vi "ADS1015 Config Formatter.vi"(11 "ADS1015 Config Options":T1 {"Comparator Queue & Disable" items=["Assert after one conversion", "Assert after two conversions", "Assert after four conversions", "Comparator disabled"]; "Latching Comparator" items=["Non-latching", "Latching"]; "Comparator Polarity" items=["Active Low", "Active High"]; "Comparator Mode" items=["Traditional Comparator w/ hysteresis", "Window Comparator"]; "Sampling Rate" items=["128SPS", "250SPS", "490SPS", "920SPS", "1600SPS", "2400SPS", "3300SPS"]; "Sampling Mode" items=["Continuous Conversion", "Single-shot (Low Power)"]; "Expected Range (Programmable Gain Amplifier)" items=["+/-6.144V", "+/-4.096V", "+/-2.048V", "+/-1.024V", "+/-0.512V", "+/-0.256V"]; "Channel" items=["Differential: Ch 0&1", "Differential: Ch 0&3", "Differential: Ch 1&3", "Differential: Ch 2&3", "Single Ended: Ch 0", "Single Ended: Ch 1", "Single Ended: Ch 2", "Single Ended: Ch 3"]}) -> (3 "Config Command":u16=4096 format="%.0x")   [LabVIEW 2014]
uses:
  ADS1015 Config Options.ctl
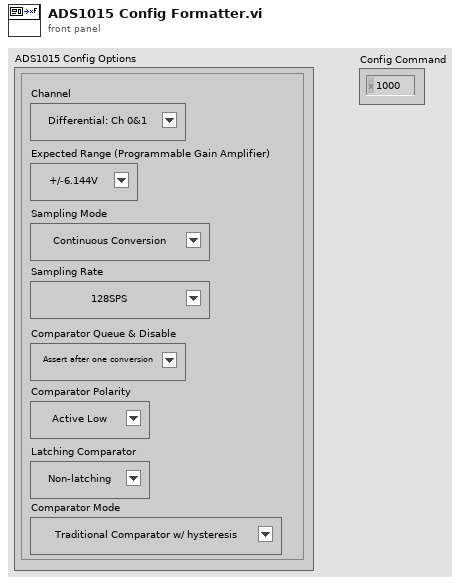
[diagram p1: front panel]
types:
  T1 = typedef "ADS1015 Config Options.ctl" = cluster{"Channel":u8, "Expected Range (Programmable Gain Amplifier)":u8, "Sampling Mode":u8, "Sampling Rate":u8, "Comparator Mode":u8, "Comparator Polarity":u8, "Latching Comparator":u8, "Comparator Queue & Disable":u8}
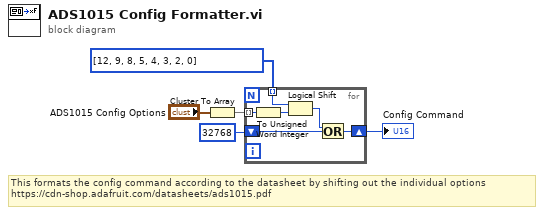
[diagram p0: block diagram]
diagram:
  # "This formats the config command according to the datasheet by shifting out the individual options\nhttps://cdn-shop.adafruit.com/datasheets/ads1015.pdf"
  n1 = Cluster To Array(cluster="ADS1015 Config Options") -> (array=w4:u8[])
  n2 = for {
    tunnel: w4 -> [w11] mode=indexing
    tunnel: i16[] [12, 9, 8, 5, 4, 3, 2, 0] -> [w10] mode=indexing
    shift-right: [w8] -> w1
    shift-left: u16 32768 -> [w7]
    n3 = To Unsigned Word Integer(number=w11) -> (unsigned 16bit integer=w6:u16)
    n4 = Logical Shift(y=w10, x=w6) -> (x << y=w9:u16)
    n5 = Or(x=w9, y=w7) -> (x .or. y?=w8:u16)
  }
  "Config Command" <- w1
